vi "Value Prompt UI.vi"(4 "Max":dbl=inf, 6 "Min":dbl=-inf, 7 "Display Format":string="%.4f", 10 "Default":dbl, 11 "Prompt":string="Enter new value") -> (1 "Cancelled":bool, 2 "New Value":dbl)   [LabVIEW 2020, in "VolatusGUIElements.lvlib" / "DblPopupControl.lvclass"]
uses:
  DblPopupControl.lvclass
  <vilib>/Utility/miscctls.llb/LVSelectionTypeDef.ctl
panel:
  in  "Abort Accept":bool
  in  "Cancel":bool
  in  "Accept":bool
  out "Prompt Display":string="Enter new value for\nDuration_s"
  in  "Value":dbl format="%.4f"
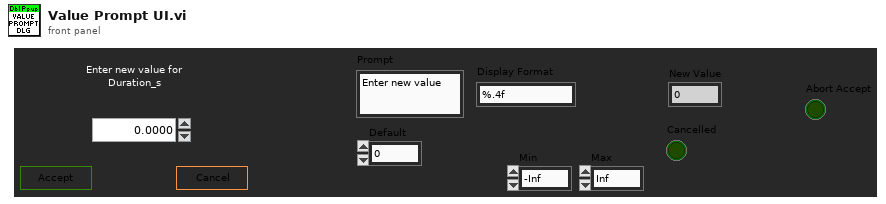
[diagram p1: front panel]
types:
  T1 = typedef "LVSelectionTypeDef.ctl" = cluster{"Selection Start":u32, "Selection End":u32}
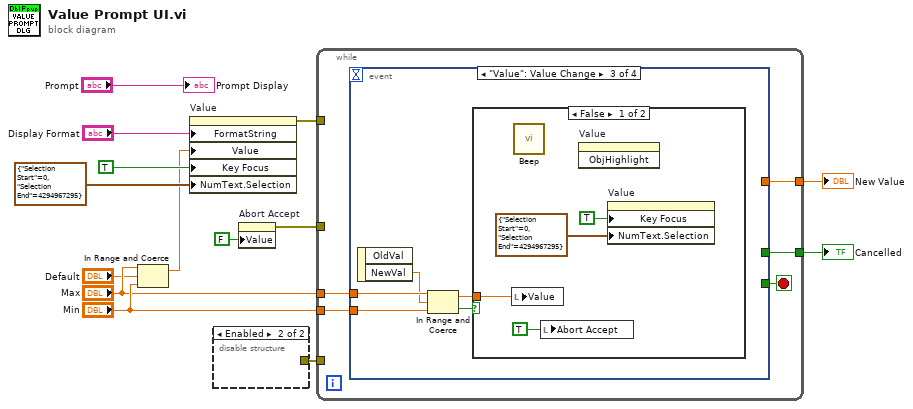
[diagram p0: block diagram]
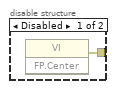
[diagram p2: hidden frame]
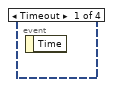
[diagram p3: hidden frame]
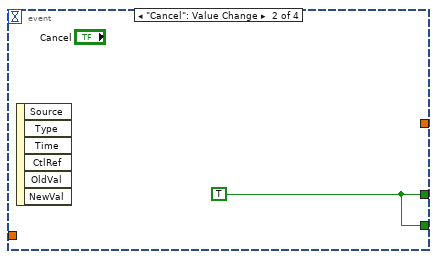
[diagram p4: hidden frame]
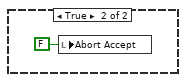
[diagram p5: hidden frame]
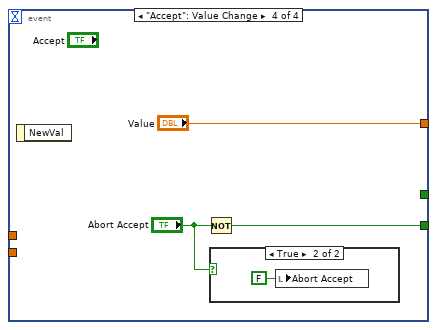
[diagram p6: hidden frame]
diagram:
  n1 = In Range and Coerce(upper limit="Max", x="Default", lower limit="Min") -> (coerced(x)=w4:dbl)  [unwired: 1 out]
  n2 = property on="Value" class="DigNum (strict)"("FormatString"="Display Format", "Value"=w4, "Key Focus"=TRUE, "NumText.Selection"=T1 {"Selection Start"=0, "Selection End"=4294967295} ("Numeric Text.Selection")) -> (error out=w8:errorcluster)  [unwired: 2 in, 1 out]
  n3 = disable-structure shown="Enabled" {
    disable-tunnel: [w15 _] -> w12
    frame Disabled {
      n4 = invoke on="Invoke Node" class="VI" method="FP.Center"() -> (error out=w15:errorcluster)  [unwired: 3 in, 2 out]
    }
    frame Enabled {
    }
  }
  n5 = property on="Abort Accept" class="Bool (strict)"("Value"=FALSE ("Abort Accept")) -> (error out=w2:errorcluster)  [unwired: 2 in, 1 out]
  n6 = while {
    tunnel: w12 -> [_]
    tunnel: [w20] -> w10
    tunnel: "Max" -> [w18]
    tunnel: "Min" -> [w17]
    tunnel: w8 -> [_]
    tunnel: [w16] -> w3
    tunnel: w2 -> [_]
    stop <- w19 stop-if-true
    n7 = event shown="[2] \"Value\": Value Change" {
      selector: _ -> [_ _ _ _]
      dyn-events: _ -> [_ _ _ _]
      timeout: _ -> [_ _ _ _]
      tunnel: [_ w21 _ _] -> w20
      tunnel: [_ w21 _ w33] -> w19
      tunnel: w18 -> [_ _ w26 _]
      tunnel: w17 -> [_ _ w25 _]
      tunnel: [_ _ _ "Value"] -> w16
      event Timeout {
        n8 = event-data() -> ()  [unwired: 1 in, 1 out]
      }
      event "Cancel": Value Change {
        w21 = TRUE
        n9 = event-data() -> ()  [unwired: 1 in, 6 out]
      }
      event "Value": Value Change {
        n10 = event-data() -> ("NewVal"=w24:dbl)  [unwired: 1 in, 1 out]
        n11 = In Range and Coerce(upper limit=w26, x=w24, lower limit=w25) -> (coerced(x)=w22:dbl, In Range?=w23:bool)
        n12 = case shown="False" w23 {
          tunnel: w22 -> [w30 _]
          frame False {
            n13 = local write "Value"(w30) -> ()
            n14 = call <vilib>:"Beep.vi"() -> ()  [unwired: 12 in]
            n15 = local write "Abort Accept"(TRUE ("Abort Accept")) -> ()
            n16 = invoke on="Value" class="DigNum (strict)" method="ObjHighlight"() -> ()  [unwired: 3 in, 3 out]
            n17 = property on="Value" class="DigNum (strict)"("Key Focus"=TRUE, "NumText.Selection"=T1 {"Selection Start"=0, "Selection End"=4294967295} ("Numeric Text.Selection")) -> ()  [unwired: 2 in, 2 out]
          }
          frame True {
            n18 = local write "Abort Accept"(FALSE ("Abort Accept")) -> ()
          }
        }
      }
      event "Accept": Value Change {
        n19 = event-data() -> ()  [unwired: 1 in, 1 out]
        n20 = Not(x="Abort Accept") -> (.not. x?=w33:bool)
        n21 = case shown="True" "Abort Accept" {
          frame False {
          }
          frame True {
            n22 = local write "Abort Accept"(FALSE ("Abort Accept")) -> ()
          }
        }
      }
    }
  }
  "New Value" <- w3
  "Cancelled" <- w10
  "Prompt Display" <- "Prompt"
